vi "Drive Controller.vi"(8 "error in":errorcluster) -> ()   [LabVIEW 2017]
doc: "This VI executes continuously carrying out the current operation and responding to updates or new operation requests. It will often contain the timing or control code that is difficult to place directly in TeleOp. This VI generally opens all sensors and motors and isolates the rest of the robot code from knowing implementation details of how the operations are carried out."
uses:
  <vilib>/Rock Robotics/WPI/Framework/Completion Status.ctl
  Drive Setpoints.ctl
  Drive Operations.ctl
  <vilib>/Rock Robotics/WPI/SafetyOutput/WPI_SafetyOutputConfigMenu.ctl
  <vilib>/Rock Robotics/SystemInterfaces/DIO/FPGA_DIOPWMChannel.ctl
  <vilib>/Rock Robotics/SystemInterfaces/DIO/FPGA_DIOChannel.ctl
  <vilib>/Rock Robotics/WPI/RobotDrive/WPI_RobotDriveOpen4MotorWithJaguar.vi
  <vilib>/Rock Robotics/WPI/Counter/WPI_CounterDigitalInputToDigitalSource.vi
panel:
  in  "Interactive Values":T1
  in  "Buttons":cluster{"Execute Cmd":bool, "Abort Cmd":bool}
  out "Command Timing":cluster{"Start Time (ms)":u32, "Iterations":i32}
  out "Status":T3
  out "Setpoints":T4(graph)
  out "Current\nCmd":string
  # "Tip: The graph shows the motor setpoints. It may also be helpful to observe inputs and sensor values.\nYou may also want to display tuning or debugging controls."
  # "Interactive Command: You may fill in the settings for a command\nand schedule it with the Execute button. You can observe and abort\nany command while fine tuning the code for the controller."
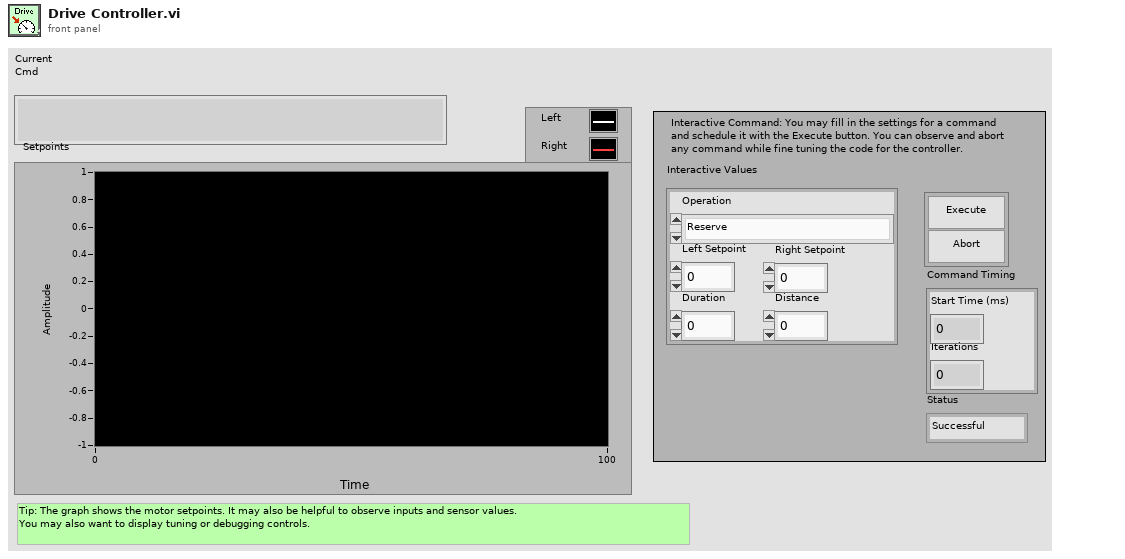
[diagram p1: front panel]
types:
  T1 = typedef "Drive Setpoints.ctl" = cluster{"Operation":T2, "Left Setpoint":dbl, "Right Setpoint":dbl, "Duration":dbl, "Distance":dbl}
  T2 = typedef "Drive Operations.ctl" = enum16{"Reserve", "Read Current", "Immediate", "Drive for Time", "Drive for Distance"}
  T3 = typedef "Completion Status.ctl" = enum16{"Successful", "Aborted", "Incomplete"}
  T4 = cluster{"Left Setpoint":dbl, "Right Setpoint":dbl}
  T5 = typedef "FPGA_DIOChannel.ctl" = enum8{"DIO 0", "DIO 1", "DIO 2", "DIO 3", "DIO 4", "DIO 5", "DIO 6", "DIO 7", "DIO 8", "DIO 9", "DIO MXP 0", "DIO MXP 1", "DIO MXP 2", "DIO MXP 3", "DIO MXP 4", "DIO MXP 5", "DIO MXP 6", "DIO MXP 7", "DIO MXP 8", "DIO MXP 9", "DIO MXP 10", "DIO MXP 11", "DIO MXP 12", "DIO MXP 13", "DIO MXP 14", "DIO MXP 15", "SPI Port CS1", "SPI Port CS2", "SPI Port CS3", "SPI Port MISO", "SPI Port MOSI", "Invalid"}
  T6 = typedef "FPGA_DIOPWMChannel.ctl" = enum8{"PWM 0", "PWM 1", "PWM 2", "PWM 3", "PWM 4", "PWM 5", "PWM 6", "PWM 7", "PWM 8", "PWM 9", "PWM MXP 0", "PWM MXP 1", "PWM MXP 2", "PWM MXP 3", "PWM MXP 4", "PWM MXP 5", "PWM MXP 6", "PWM MXP 7", "PWM MXP 8", "PWM MXP 9", "Invalid"}
  T7 = typedef "WPI_SafetyOutputConfigMenu.ctl" = enum16{"Enable", "Disable"}
  T8 = typedef "WPI_RobotDriveDevRef.ctl" = cluster{"DevStatus":errorcluster, "Motors[]":T9[], "Square Inputs":bool, "Max Output":dbl}
  T9 = typedef "WPI_MotorControlDeviceRef.ctl" = cluster{"DeviceStatus":errorcluster, "Type":T10, "PWM":cluster{"PWM Channel":T6, "DeadBand":T11}, "CAN":cluster{"Device Number":u8, "SetOutput VI Ref":variant, "GetOutput VI Ref":variant, "Enable VI Ref":variant, "Disable VI Ref":variant, "Data":variant}, "Invert":bool, "DIO PWM":cluster{"PWM \"Enable\" Channel":T6, "DIOChannel":T5, "PWM Rate":dbl}}
  T10 = typedef "WPI_MotorControlType.ctl" = enum16{"PWM", "CAN", "DIO PWM"}
  T11 = typedef "WPI_PWMDeadband.ctl" = cluster{"Name":string, "maxPositivePwm":i32, "minPositivePwm":i32, "centerPwm":i32, "maxNegativePwm":i32, "minNegativePwm":i32, "angularRange":u16}
  T12 = typedef "Command Status Info.ctl" = cluster{"Name":string, "Status":T3, "notifier out":T13}
  T13 = typedef "Completion Notifier.ctl" = refnum<notifier>
  T14 = cluster{"SubSystem Data":T1, cluster{"Start Time (ms)":u32, "Iterations":i32}, cluster{"Command Info":T12, "Description":string, "Default Command":T1, "queue out":refnum<queue>, "Subsystem Name":string}}
  T15 = typedef "WPI_DigitalInputDevRef.ctl" = cluster{"DevStatus":errorcluster, "DIO Channel":T5}
  T16 = typedef "FPGA_CounterEncoderSourceConvertionLVSourceType.ctl" = cluster{"DevStatus":errorcluster, "AnalogTriggerMode?":bool, "DigitalMode":cluster{"DIO Channel":T17}, "AnalogTriggerMode":cluster{"AnalogTriggerIndex":T18, "OutputType":T19}}
  T17 = typedef "FPGA_DIODigitalSourceChannel.ctl" = enum8{"DIO 0", "DIO 1", "DIO 2", "DIO 3", "DIO 4", "DIO 5", "DIO 6", "DIO 7", "DIO 8", "DIO 9", "DIO MXP 0", "DIO MXP 1", "DIO MXP 2", "DIO MXP 3", "DIO MXP 4", "DIO MXP 5", "DIO MXP 6", "DIO MXP 7", "DIO MXP 8", "DIO MXP 9", "DIO MXP 10", "DIO MXP 11", "DIO MXP 12", "DIO MXP 13", "DIO MXP 14", "DIO MXP 15", "Disabled"}
  T18 = typedef "FPGA_AnalogTriggerIndex.ctl" = enum8{"Trig 0", "Trig 1", "Trig 2", "Trig 3", "Trig 4", "Trig 5", "Trig 6", "Trig 7", "Invalid"}
  T19 = typedef "FPGA_AnalogTriggerOutType.ctl" = enum16{"InWindow", "TriggerState", "Rising", "Falling"}
  T20 = typedef "WPI_EncoderDevRef.ctl" = cluster{"DevStatus":errorcluster, "EncoderIndex":T21, "CounterIndex":T22, "DistancePerCount":dbl, "Decoding Type":T23}
  T21 = typedef "FPGA_EncoderIdx.ctl" = enum8{"Enc 0", "Enc 1", "Enc 2", "Enc 3", "Enc 4", "Enc 5", "Enc 6", "Enc 7", "Invalid"}
  T22 = typedef "FPGA_CounterCtrSystemIndex.ctl" = enum8{"Ctr 0", "Ctr 1", "Ctr 2", "Ctr 3", "Ctr 4", "Ctr 5", "Ctr 6", "Ctr 7", "Invalid"}
  T23 = typedef "WPI_EncoderType.ctl" = enum16{"1x", "2x", "4x"}
  T24 = cluster{"SubSystem Data":T1, cluster{"Start Time (ms)":u32, "Iterations":i32}, "Default Command Arguments":cluster{"Command Info":T12, "Description":string, "Default Command":T1, "queue out":refnum<queue>, "Subsystem Name":string}}
  T25 = cluster{"Don't move motors while reserved":dbl, "Don't move motors while reserved":dbl}
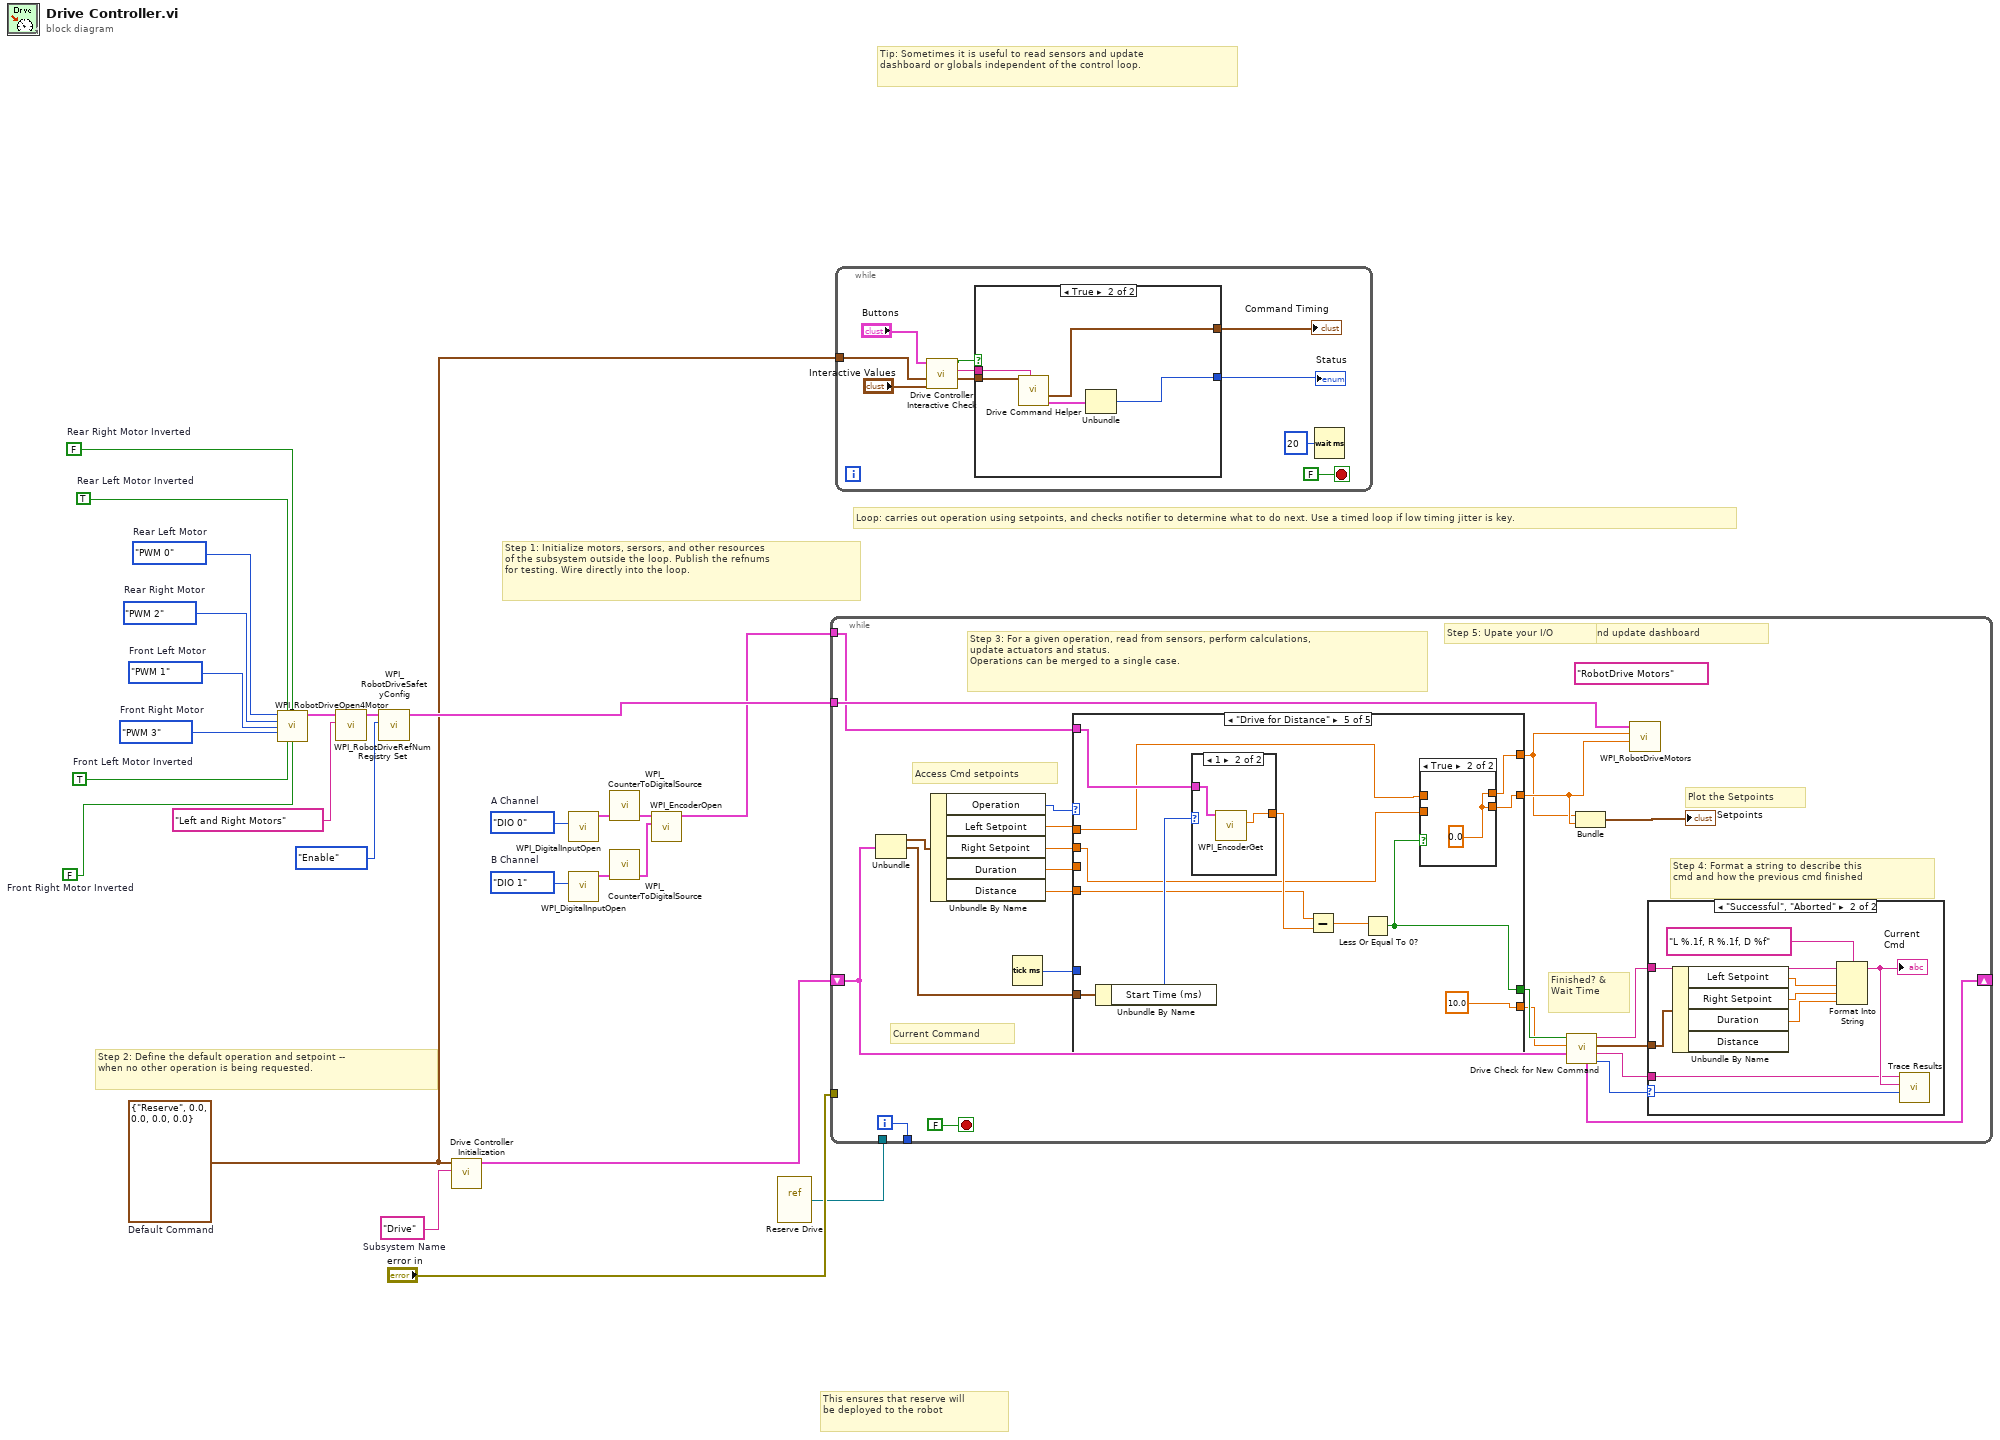
[diagram p0: block diagram]
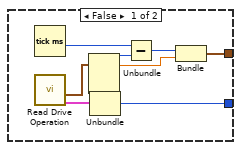
[diagram p2: hidden frame]
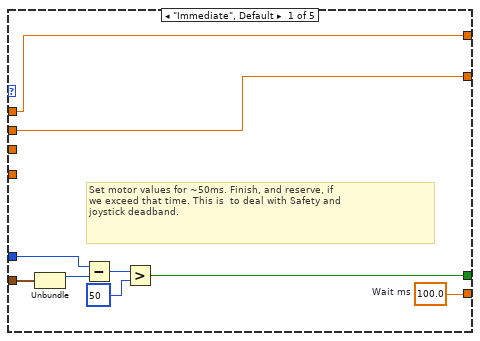
[diagram p3: hidden frame]
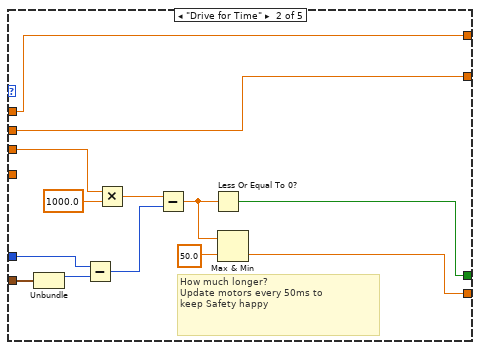
[diagram p4: hidden frame]
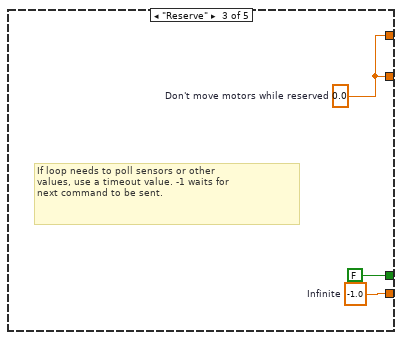
[diagram p5: hidden frame]
diagram:
  w1 = FPGA_DIOChannel."DIO 1"  # B Channel
  w4 = FPGA_DIOChannel."DIO 0"  # A Channel
  w8 = TRUE  # Front Left Motor Inverted
  w9 = FALSE  # Front Right Motor Inverted
  w10 = FALSE  # Rear Right Motor Inverted
  w11 = TRUE  # Rear Left Motor Inverted
  w12 = FPGA_DIOPWMChannel."PWM 2"  # Rear Right Motor
  w13 = FPGA_DIOPWMChannel."PWM 3"  # Front Right Motor
  w14 = FPGA_DIOPWMChannel."PWM 0"  # Rear Left Motor
  w15 = FPGA_DIOPWMChannel."PWM 1"  # Front Left Motor
  w17 = T1 {"Operation"=enum."Reserve", "Left Setpoint"=0.0, "Right Setpoint"=0.0, "Duration"=0.0, "Distance"=0.0}  # Default Command
  w25 = "Drive"  # Subsystem Name
  # "Step 2: Define the default operation and setpoint --\nwhen no other operation is being requested."
  # "This ensures that reserve will\nbe deployed to the robot"
  # "Tip: Sometimes it is useful to read sensors and update\ndashboard or globals independent of the control loop."
  # "Step 1: Initialize motors, sersors, and other resources\nof the subsystem outside the loop. Publish the refnums\nfor testing. Wire directly into the loop."
  # "Loop: carries out operation using setpoints, and checks notifier to determine what to do next. Use a timed loop if low timing jitter is key."
  n1 = call-poly <vilib>:"WPI_RobotDriveOpen4Motor.vi"("Rear Left Motor"=w14, "Rear Left Motor Inverted"=w11, "Rear Right Motor Inverted"=w10, "Rear Right Motor"=w12, "Front Left Motor"=w15, "Front Right Motor"=w13, "Front Left Motor Inverted"=w8, "Front Right Motor Inverted"=w9) -> ("RobotDriveDevRef"=w16:T8)  [unwired: 6 in, 1 out]
  n2 = call <vilib>:"WPI_RobotDriveRefNum Registry Set.vi"("refnum name"="Left and Right Motors", "RobotDriveDevRef"=w16) -> ("RobotDriveDevRef"=w23:T8)  [unwired: 2 in, 7 out]
  n3 = call <vilib>:"WPI_RobotDriveSafetyConfig.vi"("mode"=WPI_SafetyOutputConfigMenu."Enable", "RobotDriveDevRef"=w23) -> ("RobotDriveDevRef"=w21:T8)  [unwired: 8 in, 1 out]
  n4 = call "Drive Controller Initialization.vi"("Subsystem Name"=w25, "Default Command"=w17) -> ("Current Command"=w19:T14)  [unwired: 9 in]
  n5 = call <vilib>:"WPI_DigitalInputOpen.vi"("DIO Channel"=w4) -> ("DigitalInputDevRef"=w5:T15)  [unwired: 1 in, 9 out]
  n6 = call <vilib>:"WPI_DigitalInputOpen.vi"("DIO Channel"=w1) -> ("DigitalInputDevRef"=w2:T15)  [unwired: 1 in, 9 out]
  n7 = call-poly <vilib>:"WPI_CounterToDigitalSource.vi"("DigitalInputDevRef"=w5) -> ("Digital Source"=w6:T16)  [unwired: 6 out]
  n8 = call-poly <vilib>:"WPI_CounterToDigitalSource.vi"("DigitalInputDevRef"=w2) -> ("Digital Source"=w3:T16)  [unwired: 6 out]
  n9 = call <vilib>:"WPI_EncoderOpen.vi"("BSource"=w3, "ASource"=w6) -> ("EncoderDevRef"=w7:T20)  [unwired: 6 in, 3 out]
  n10 = vi-ref "Reserve Drive.vi"() -> (w18:refnum<vi>)
  n11 = while {
    shift-right: [w42] -> _
    shift-left: w19 -> [w37]
    tunnel: [w47] -> _
    tunnel: w21 -> [w45]
    tunnel: "error in" -> [_]
    tunnel: w18 -> [_]
    tunnel: w7 -> [w34]
    i -> [w47]
    stop <- FALSE stop-if-true
    (unwired) "RobotDrive Motors" ("Name")
    # "Step 5: Upate your I/O"
    # "Step 4: Format a string to describe this\ncmd and how the previous cmd finished"
    # "Current Command"
    # "Update motors and update dashboard"
    # "Plot the Setpoints"
    # "Access Cmd setpoints"
    # "Finished? &\nWait Time"
    # "Step 3: For a given operation, read from sensors, perform calculations,\nupdate actuators and status.\nOperations can be merged to a single case."
    n12 = Unbundle(w37) -> ("SubSystem Data"=w28:T1, w38:cluster{"Start Time (ms)":u32, "Iterations":i32})  [unwired: 1 out]
    n13 = Unbundle By Name(w28) -> ("Operation"=w33:T2, "Left Setpoint"=w32:dbl, "Right Setpoint"=w31:dbl, "Duration"=w30:dbl, "Distance"=w29:dbl)
    n14 = Tick Count (ms)() -> (millisecond timer value=w44:u32)
    n15 = case shown="\"Drive for Distance\"" w33 {
      tunnel: w38 -> [w53 w67 _ _ w80]
      tunnel: w32 -> [w51 w61 _ _ w76]
      tunnel: w31 -> [w50 w60 _ _ w77]
      tunnel: w30 -> [_ w65 _ _ _]
      tunnel: w44 -> [w54 w64 _ _ _]
      tunnel: [w52 w59 FALSE ("ignore previous (F)") _ w85] -> w36
      tunnel: [w51 w61 w71 _ w75] -> w26
      tunnel: [w50 w60 w71 _ w74] -> w27
      tunnel: w34 -> [_ _ _ _ w82]
      tunnel: w29 -> [_ _ _ _ w79]
      tunnel: [w49 w58 w72 _ 10.0 ("Infinite")] -> w35
      frame "Immediate", Default {
        w49 = 100.0  # Wait ms
        # "Set motor values for ~50ms. Finish, and reserve, if\nwe exceed that time. This is  to deal with Safety and\njoystick deadband."
        n16 = Unbundle(w53) -> ("Start Time (ms)"=w55:u32)  [unwired: 1 out]
        n17 = Subtract(x=w54, y=w55) -> (x-y=w56:u32)
        n18 = Greater?(x=w56, y=u8 50 ("Left Motor")) -> (0:w52:bool)
      }
      frame "Drive for Time" {
        # "How much longer?\nUpdate motors every 50ms to\nkeep Safety happy"
        n19 = Unbundle(w67) -> ("Start Time (ms)"=w66:u32)  [unwired: 1 out]
        n20 = Subtract(x=w64, y=w66) -> (x-y=w70:u32)
        n21 = Multiply(x=w65, y=1000.0) -> (x*y=w69:dbl)
        n22 = Subtract(x=w69, y=w70) -> (x-y=w63:dbl)
        n23 = Less Or Equal To 0?(x=w63) -> (x <= 0?=w59:bool)
        n24 = Max & Min(x=w63, y=50.0) -> (min(x,y)=w58:dbl)  [unwired: 1 out]
      }
      frame "Reserve" {
        w71 = 0.0  # Don't move motors while reserved
        w72 = -1.0  # Infinite
        # "If loop needs to poll sensors or other\nvalues, use a timeout value. -1 waits for\nnext command to be sent."
      }
      frame "Read Current" {
      }
      frame "Drive for Distance" {
        n25 = Unbundle By Name(w80) -> ("Start Time (ms)"=w81:u32)
        n26 = case shown="1" w81 {
          tunnel: w82 -> [_ w87]
          tunnel: [_ w86] -> w83
          frame 0, Default {
          }
          frame 1 {
            n27 = call <vilib>:"WPI_EncoderGet.vi"("EncoderDevRef"=w87) -> ("Distance"=w86:dbl)  [unwired: 5 in, 5 out]
          }
        }
        n28 = Subtract(x=w79, y=w83) -> (x-y=w84:dbl)
        n29 = Less Or Equal To 0?(x=w84) -> (x <= 0?=w85:bool)
        n30 = case shown="True" w85 {
          tunnel: [_ w88] -> w74
          tunnel: w76 -> [_ _]
          tunnel: w77 -> [_ _]
          tunnel: [_ w88] -> w75
          frame False {
          }
          frame True {
            w88 = 0.0
          }
        }
      }
    }
    n31 = call "Drive Check for New Command.vi"("input cluster"=w37, "Wait time (ms)"=w35, "Finished?"=w36) -> ("Completion"=w43:T3, "Subsystem Name"=w39:string, "Current Command"=w40:T1, "Initial Trace String"=w41:string, "Next Command"=w42:T24)  [unwired: 4 in]
    n32 = Bundle("Don't move motors while reserved"=w26, "Don't move motors while reserved"=w27) -> (→"Setpoints":T25)  [unwired: 1 in]
    n33 = call <vilib>:"WPI_RobotDriveMotors.vi"("RightSpeed"=w27, "LeftSpeed"=w26, "RobotDriveDevRef"=w45) -> ()  [unwired: 1 in, 8 out]
    n34 = case shown="\"Successful\", \"Aborted\"" w43 {
      selector: w43 -> [_ w97]
      tunnel: w41 -> [_ w95]
      tunnel: w40 -> [_ w92]
      tunnel: w39 -> [_ w93]
      frame "Incomplete", Default {
        # "Continuing current command"
      }
      frame "Successful", "Aborted" {
        # "Report and setup for next command"
        n35 = Unbundle By Name(w92) -> ("Left Setpoint"=w91:dbl, "Right Setpoint"=w90:dbl, "Duration"=w89:dbl)  [unwired: 1 out]
        n36 = Format Into String(format string="L %.1f, R %.1f, D %f", initial string=w95, w91, w90, w89) -> (resulting string=w94:string)  [unwired: 1 in, 1 out]
        "Current\nCmd" <- w94
        n37 = call <vilib>:"Trace Results.vi"("Status of previous command"=w97, "Description"=w94, "Subsystem"=w93) -> ()  [unwired: 9 in]
      }
    }
  }
  n38 = while {
    tunnel: w17 -> [w99]
    stop <- FALSE stop-if-true
    n39 = call "Drive Controller Interactive Check.vi"("Interactive Command In"="Interactive Values", "Default Command"=w99, "Buttons"="Buttons") -> ("Interactive Command Out"=w101:T1, "Trace String"=w102:string, "Schedule"=w103:bool)  [unwired: 6 in]
    n40 = case shown="True" w103 {
      tunnel: [w112 w120] -> w104
      tunnel: [w111 w116] -> w105
      tunnel: w102 -> [_ w118]
      tunnel: w101 -> [_ w117]
      frame False {
        n41 = Tick Count (ms)() -> (millisecond timer value=w115:u32)
        n42 = call "Read Drive Operation.vi"() -> ("Command Info"=w109:T12, "SubSystem Data"=w108:T1)  [unwired: 9 in, 1 out]
        n43 = Unbundle(w108) -> ("Operation"=w113:T2, "Left Setpoint"=w110:dbl)  [unwired: 3 out]
        n44 = Unbundle(w109) -> ("Status"=w112:T3)  [unwired: 2 out]
        n45 = Subtract(x=w115, y=w113) -> (x-y=w114:u32)
        n46 = Bundle(w114, "Left Setpoint"=w110) -> (w111:cluster{u32, "Left Setpoint":dbl})  [unwired: 1 in]
      }
      frame True {
        n47 = call "Drive Command Helper.vi"("Description"=w118, "SubSystem Data"=w117) -> ("Command Info Out"=w119:T12, "Command Timing"=w116:cluster{"Start Time (ms)":u32, "Iterations":i32})  [unwired: 7 in, 1 out]
        n48 = Unbundle(w119) -> ("Status"=w120:T3)  [unwired: 2 out]
      }
    }
    "Status" <- w104
    "Command Timing" <- w105
    n49 = Wait (ms)(milliseconds to wait=u32 20) -> ()  [unwired: 1 out]
  }
